vi "Simple Sine Waveform.vi"(5 "n points":i32=100, 6 "delta t":dbl=1.0, 7 "amplitude":dbl=1.0, 9 "n cycles":dbl=1.0, 10 "t0":dbl=-1.0, 11 "offset":dbl) -> (3 "sine waveform":waveform(dbl))   [LabVIEW 2015]
doc: "Produces a sine wave."
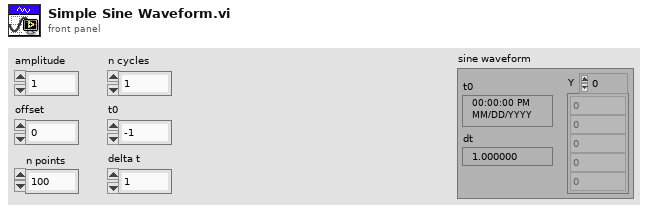
[diagram p1: front panel]
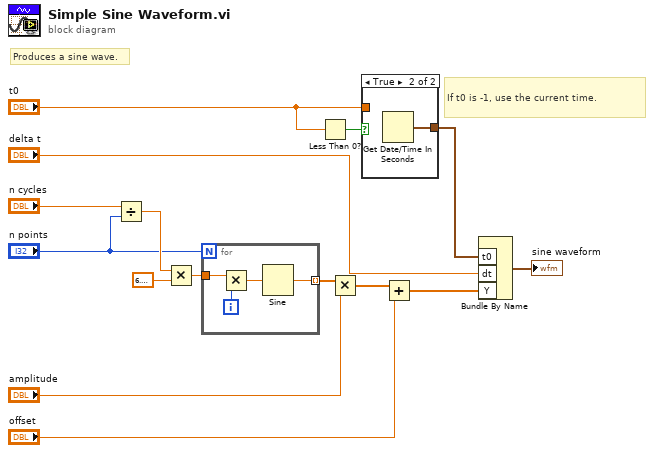
[diagram p0: block diagram]
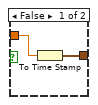
[diagram p2: hidden frame]
diagram:
  # "If t0 is -1, use the current time."
  # "Produces a sine wave."
  n1 = Divide(x="n cycles", y="n points") -> (x/y=w7:dbl)
  n2 = Multiply(x=w7, y=6.283185307179586) -> (x*y=w5:dbl)
  n3 = for {
    N: "n points" -> [_]
    tunnel: [w19] -> w13 mode=indexing
    tunnel: w5 -> [w16]
    i -> [w17]
    n4 = Multiply(x=w16, y=w17) -> (x*y=w18:dbl)
    n5 = Sine(x=w18) -> (sin(x)=w19:dbl)
  }
  n6 = Less Than 0?(x="t0") -> (x < 0?=w1:bool)
  n7 = Multiply(x=w13, y="amplitude") -> (x*y=w11:dbl[])
  n8 = case shown="True" w1 {
    tunnel: [w21 w22] -> w3
    tunnel: "t0" -> [w20 _]
    frame False {
      n9 = To Time Stamp(1:w20) -> (0:w21:timestamp)
    }
    frame True {
      n10 = Get Date/Time In Seconds() -> (seconds since 1Jan1904=w22:timestamp)
    }
  }
  n11 = Add(x=w11, y="offset") -> (x+y=w9:dbl[])
  n12 = Bundle By Name("t0"=w3, "dt"="delta t", "Y"=w9) -> (→"sine waveform":waveform(dbl))  [unwired: 1 out]
